vi "TestMain.vi"() -> ()   [LabVIEW 2019]
uses:
  <vilib>/Platform/TimedLoop/XDataNode/timing_clust.ctl
  <vilib>/Platform/TimedLoop/XDataNode/nitl_modes.ctl
  <vilib>/Platform/TimedLoop/XDataNode/wakeup.ctl
  <vilib>/myRIO/Instrument Drivers/Onboard IO/PWM/typedefs/PWM Reference.ctl
  <vilib>/myRIO/Common/Instrument Driver Framework/Utilities/typedefs/myRIO Generic Hardware Reference.ctl
  <vilib>/myRIO/Common/Instrument Driver Framework/Utilities/typedefs/Hardware Version Enum.ctl
  <vilib>/myRIO/Common/Instrument Driver Framework/Utilities/typedefs/myRIO v1.0 Reference.ctl
  <vilib>/myRIO/Common/Instrument Driver Framework/Utilities/typedefs/Generic FPGA Reference.ctl
  <vilib>/myRIO/Common/Instrument Driver Framework/myRIO v1.0/PWM/typedefs/PWM Channels Enum.ctl
  <vilib>/myRIO/Instrument Drivers/Onboard IO/PWM/typedefs/PWM Configuration.ctl
  <vilib>/userdefined/High Color/nirio_resource_hc.ctl
  <vilib>/myRIO/Instrument Drivers/Onboard IO/DIO/typedefs/DIO Reference.ctl
  <vilib>/myRIO/Common/Instrument Driver Framework/myRIO v1.0/DIO/typedefs/DIO Channels List.ctl
  <vilib>/myRIO/Common/Instrument Driver Framework/myRIO v1.0/DIO/typedefs/DIO Channels Enum.ctl
  <vilib>/myRIO/Common/Instrument Driver Framework/Utilities/vis/Is FPGA Ref Available.vi
  <vilib>/myRIO/Common/Instrument Driver Framework/myRIO v1.0/PWM/vis/myRIO v1.1 Open PWM.vi
  <vilib>/myRIO/Instrument Drivers/Onboard IO/PWM/vis/Set Duty Cycle and Frequency.vi
  <vilib>/myRIO/Common/Instrument Driver Framework/myRIO v1.0/DIO/vis/myRIO v1.1 Open DIO.vi
  <extravilib>/ChannelInstances/Tag-bool/Write With Abort.vi
  <extravilib>/ChannelInstances/Tag-bool/Read With Abort.vi
  <vilib>/myRIO/Common/Instrument Driver Framework/Utilities/vis/Validate Channels.vi
  <vilib>/myRIO/Common/Instrument Driver Framework/myRIO v1.0/PWM/vis/myRIO v1.0 Reserve PWM.vi
  <vilib>/myRIO/Common/Instrument Driver Framework/myRIO v1.0/DIO/vis/myRIO v1.0 Reserve DIO.vi
  <vilib>/myRIO/Common/Instrument Driver Framework/myRIO v1.0/I2C/vis/myRIO v1.0 Close I2C.vi
  <vilib>/myRIO/Common/Instrument Driver Framework/myRIO v1.0/UART/vis/myRIO v1.0 Close UART.vi
  <vilib>/myRIO/Common/Instrument Driver Framework/myRIO v1.0/PWM/vis/myRIO v1.0 Build MUX Configuration PWM.vi
  <vilib>/myRIO/Common/Instrument Driver Framework/myRIO v1.0/Resource Manager/vis/myRIO v1.0 Reserve Channel List.vi
  <vilib>/myRIO/Common/Instrument Driver Framework/myRIO v1.0/DIO/vis/myRIO v1.0 Build MUX Configuration DIO.vi
  <vilib>/myRIO/Common/Instrument Driver Framework/myRIO v1.0/I2C/vis/myRIO v1.0 Unreserve I2C.vi
  <vilib>/myRIO/Common/Instrument Driver Framework/myRIO v1.0/Resource Manager/vis/myRIO v1.0 Create Configuration List.vi
  <vilib>/myRIO/Common/Instrument Driver Framework/myRIO v1.0/Resource Manager/vis/myRIO v1.0 Reserve Channel.vi
  <vilib>/myRIO/Common/Instrument Driver Framework/myRIO v1.0/Resource Manager/vis/myRIO v1.0 Unreserve Channel.vi
  <vilib>/myRIO/Common/Instrument Driver Framework/myRIO v1.0/I2C/vis/myRIO v1.0 Build MUX Configuration I2C.vi
  <vilib>/myRIO/Common/Instrument Driver Framework/myRIO v1.0/Resource Manager/vis/myRIO v1.0 Unreserve Channel List.vi
  <vilib>/myRIO/Common/Instrument Driver Framework/myRIO v1.0/Resource Manager/vis/myRIO v1.0 Build Mutex Name.vi
  <vilib>/Instr/_visa.llb/VISA Configure Serial Port (Instr).vi
  <extravilib>/ChannelInstances/Tag-bool/Instantiate.vi
  <extravilib>/ChannelInstances/Tag-bool/EndpointRead.vi
  <vilib>/Utility/VariantDataType/GetNumericInfo.vi
  <vilib>/Utility/error.llb/Error Cluster From Error Code.vi
  <vilib>/myRIO/Common/Instrument Driver Framework/myRIO v1.0/myRIO v1.1 Open.vi
  <vilib>/myRIO/Common/Instrument Driver Framework/Utilities/vis/IO Manager.vi
  <vilib>/myRIO/Common/Instrument Driver Framework/Utilities/vis/Configuration Manager.vi
  <vilib>/myRIO/Common/Instrument Driver Framework/myRIO v1.0/Resource Manager/vis/myRIO v1.0 Configure IO.vi
  <vilib>/myRIO/Common/Instrument Driver Framework/myRIO v1.0/myRIO v1.0 Close.vi
  <vilib>/myRIO/Common/Instrument Driver Framework/myRIO v1.0/PWM/vis/myRIO v1.0 Write PWM.vi
  <vilib>/myRIO/Common/Instrument Driver Framework/myRIO v1.0/DIO/vis/myRIO v1.0 Write DIO.vi
  <vilib>/myRIO/Common/Instrument Driver Framework/myRIO v1.0/I2C/vis/myRIO v1.0 Shutdown I2C.vi
  <vilib>/rvi/errors/niLvFpgaAdjustHostInterfaceError.vi
  <vilib>/FPGAPlugInAG/Dynamic/niLvFpga_Abort_Dynamic.vi
  <vilib>/myRIO/Common/Instrument Driver Framework/Utilities/vis/FPGA Ref Manager.vi
  <vilib>/myRIO/Common/Instrument Driver Framework/myRIO v1.0/myRIO v1.0 Reset FPGA.vi
  <vilib>/myRIO/Common/Instrument Driver Framework/myRIO v1.0/IRQ/vis/myRIO v1.0 IRQ Info FGV.vi
  <vilib>/myRIO/Common/Instrument Driver Framework/myRIO v1.0/IRQ/vis/myRIO v1.0 Timer IRQ Info FGV.vi
  <vilib>/myRIO/Common/Instrument Driver Framework/myRIO v1.0/IRQ/vis/myRIO v1.0 ISR Agent.vi
  <vilib>/myRIO/Instrument Drivers/Utilities/vis/Reset Index.vi
  <vilib>/myRIO/Common/Instrument Driver Framework/myRIO v1.0/Resource Manager/vis/myRIO v1.0 Block Write Resource Manager.vi
  <vilib>/FPGAPlugInAG/Dynamic/niLvFpga_Close_Dynamic.vi
  <extravilib>/ChannelInstances/Tag-bool/Endpoint.vi
  <vilib>/platform/TimedLoop/XDataNode/XDataNode.xnode
  <vilib>/myRIO/Express VI/Onboard IO/PWM/PWM Express VI.xnode
  <vilib>/myRIO/Instrument Drivers/Onboard IO/PWM/vis/myRIO PWM Open.xnode
  <vilib>/myRIO/Express VI/Onboard IO/DO/DO Express VI.xnode
  <vilib>/myRIO/Instrument Drivers/Onboard IO/DIO/vis/myRIO DIO Open.xnode
  <vilib>/rvi/interface/nirviReadWriteControl/nirviReadWriteControl.xnode
  <vilib>/rvi/interface/nirviMethod/nirviMethod.xnode
  <vilib>/rvi/interface/nirviCloseFPGA/nirviCloseFPGA.xnode
  <vilib>/rvi/interface/Simulation/niFpgaSimulationCallBeginRW.vi
  <vilib>/Platform/TimedLoop/XDataNode/XDNodeRunTimeDep.lvlib
  <vilib>/myRIO/Instrument Drivers/Utilities/Utilities.lvlib
  NiFpgaLv.dll
  <extravilib>/ChannelInstances/Tag-bool.lvlib
  <vilib>/myRIO/Instrument Drivers/Onboard IO/PWM/PWM.lvlib
  <vilib>/myRIO/Instrument Drivers/Onboard IO/DIO/DIO.lvlib
  <vilib>/myRIO/Instrument Drivers/Onboard IO/I2C/I2C.lvlib
panel:
  in  "Log file path":path
  out "Duty Cycle":dbl
  in  "Angle limit":i32
  in  "D":dbl
  in  "I":dbl
  in  "P":dbl
  in  "RPM":u16
  out "Raw output from GPS":string
  in  "Organised Output from the GPS":T1(tab)
  out "GPGSV":string
  out "number of message":string
  out "msg1":string
  out "Satelite in view":string
  in  "Satelite_id/elevation/azimuth/SNR 17":enum32{"Msg 1", "Msg 2", "Msg 3", "Msg 4"}(tab)
  out "Satelite_id/elevation/azimuth/SNR":string[](array[string])
  out "Satelite_id/elevation/azimuth/SNR 2":string[](array[string])
  out "Satelite_id/elevation/azimuth/SNR 3":string[](array[string])
  out "Satelite_id/elevation/azimuth/SNR 4":string[](array[string])
  out "Signal ID / Check sum":string[](array[string])
  out "Signal ID / Check sum 2":string[](array[string])
  out "Satelite_id/elevation/azimuth/SNR 8":string[](array[string])
  out "Satelite_id/elevation/azimuth/SNR 7":string[](array[string])
  out "Satelite_id/elevation/azimuth/SNR 6":string[](array[string])
  out "Satelite_id/elevation/azimuth/SNR 5":string[](array[string])
  out "Signal ID / Check sum 3":string[](array[string])
  out "Satelite_id/elevation/azimuth/SNR 12":string[](array[string])
  out "Satelite_id/elevation/azimuth/SNR 11":string[](array[string])
  out "Satelite_id/elevation/azimuth/SNR 10":string[](array[string])
  out "Satelite_id/elevation/azimuth/SNR 9":string[](array[string])
  out "Signal ID / Check sum 4":string[](array[string])
  out "Satelite_id/elevation/azimuth/SNR 16":string[](array[string])
  out "Satelite_id/elevation/azimuth/SNR 15":string[](array[string])
  out "Satelite_id/elevation/azimuth/SNR 14":string[](array[string])
  out "Satelite_id/elevation/azimuth/SNR 13":string[](array[string])
  out "GLGSV 2":string
  out "number of message 2":string
  out "msg1 2":string
  out "Satelite in view 2":string
  in  "Satelite_id/elevation/azimuth/SNR 34":enum32{"Msg 1", "Msg 2", "Msg 3", "Msg 4"}(tab)
  out "Satelite_id/elevation/azimuth/SNR 21":string[](array[string])
  out "Satelite_id/elevation/azimuth/SNR 20":string[](array[string])
  out "Satelite_id/elevation/azimuth/SNR 19":string[](array[string])
  out "Satelite_id/elevation/azimuth/SNR 18":string[](array[string])
  out "Signal ID / Check sum 5":string[](array[string])
  out "Signal ID / Check sum 6":string[](array[string])
  out "Satelite_id/elevation/azimuth/SNR 25":string[](array[string])
  out "Satelite_id/elevation/azimuth/SNR 22":string[](array[string])
  out "Satelite_id/elevation/azimuth/SNR 23":string[](array[string])
  out "Satelite_id/elevation/azimuth/SNR 24":string[](array[string])
  out "Signal ID / Check sum 7":string[](array[string])
  out "Satelite_id/elevation/azimuth/SNR 29":string[](array[string])
  out "Satelite_id/elevation/azimuth/SNR 26":string[](array[string])
  out "Satelite_id/elevation/azimuth/SNR 27":string[](array[string])
  out "Satelite_id/elevation/azimuth/SNR 28":string[](array[string])
  out "Signal ID / Check sum 8":string[](array[string])
  out "Satelite_id/elevation/azimuth/SNR 33":string[](array[string])
  out "Satelite_id/elevation/azimuth/SNR 30":string[](array[string])
  out "Satelite_id/elevation/azimuth/SNR 31":string[](array[string])
  out "Satelite_id/elevation/azimuth/SNR 32":string[](array[string])
  out "GAGSV 3":string
  out "number of message 3":string
  out "msg1 3":string
  out "Satelite in view 3":string
  in  "Satelite_id/elevation/azimuth/SNR 51":enum32{"Msg 1", "Msg 2", "Msg 3", "Msg 4"}(tab)
  out "Satelite_id/elevation/azimuth/SNR 38":string[](array[string])
  out "Satelite_id/elevation/azimuth/SNR 37":string[](array[string])
  out "Satelite_id/elevation/azimuth/SNR 36":string[](array[string])
  out "Satelite_id/elevation/azimuth/SNR 35":string[](array[string])
  out "Signal ID / Check sum 9":string[](array[string])
  out "Signal ID / Check sum 10":string[](array[string])
  out "Satelite_id/elevation/azimuth/SNR 42":string[](array[string])
  out "Satelite_id/elevation/azimuth/SNR 39":string[](array[string])
  out "Satelite_id/elevation/azimuth/SNR 40":string[](array[string])
  out "Satelite_id/elevation/azimuth/SNR 41":string[](array[string])
  out "Signal ID / Check sum 11":string[](array[string])
  out "Satelite_id/elevation/azimuth/SNR 46":string[](array[string])
  out "Satelite_id/elevation/azimuth/SNR 43":string[](array[string])
  out "Satelite_id/elevation/azimuth/SNR 44":string[](array[string])
  out "Satelite_id/elevation/azimuth/SNR 45":string[](array[string])
  out "Signal ID / Check sum 12":string[](array[string])
  out "Satelite_id/elevation/azimuth/SNR 50":string[](array[string])
  out "Satelite_id/elevation/azimuth/SNR 47":string[](array[string])
  out "Satelite_id/elevation/azimuth/SNR 48":string[](array[string])
  out "Satelite_id/elevation/azimuth/SNR 49":string[](array[string])
  out "GBGSV 4":string
  out "number of message 4":string
  out "msg1 4":string
  out "Satelite in view 4":string
  in  "Satelite_id/elevation/azimuth/SNR 68":enum32{"Msg 1", "Msg 2", "Msg 3", "Msg 4"}(tab)
  out "Satelite_id/elevation/azimuth/SNR 55":string[](array[string])
  out "Satelite_id/elevation/azimuth/SNR 54":string[](array[string])
  out "Satelite_id/elevation/azimuth/SNR 53":string[](array[string])
  out "Satelite_id/elevation/azimuth/SNR 52":string[](array[string])
  out "Signal ID / Check sum 13":string[](array[string])
  out "Signal ID / Check sum 14":string[](array[string])
  out "Satelite_id/elevation/azimuth/SNR 59":string[](array[string])
  out "Satelite_id/elevation/azimuth/SNR 56":string[](array[string])
  out "Satelite_id/elevation/azimuth/SNR 57":string[](array[string])
  out "Satelite_id/elevation/azimuth/SNR 58":string[](array[string])
  out "Signal ID / Check sum 15":string[](array[string])
  out "Satelite_id/elevation/azimuth/SNR 63":string[](array[string])
  out "Satelite_id/elevation/azimuth/SNR 60":string[](array[string])
  out "Satelite_id/elevation/azimuth/SNR 61":string[](array[string])
  out "Satelite_id/elevation/azimuth/SNR 62":string[](array[string])
  out "Signal ID / Check sum 16":string[](array[string])
  out "Satelite_id/elevation/azimuth/SNR 67":string[](array[string])
  out "Satelite_id/elevation/azimuth/SNR 64":string[](array[string])
  out "Satelite_id/elevation/azimuth/SNR 65":string[](array[string])
  out "Satelite_id/elevation/azimuth/SNR 66":string[](array[string])
  out "UTC Time":string
  out "N/S":string
  out "Long":string
  out "Mode":string
  out "Status":string
  out "Lat":string
  out "Course over Ground [Degrees]":string
  out "date[ddmmyy]":string
  out "E/W":string
  out "Speed over ground[knot]":string
  out "xxRMC":string
  out "NavStatus":string
  out "Checksum":string
  out "Carriage return":string
  out "Lat 2":string
  out "NS":string
  out "GLL":string
  out "Long 3":string
  out "EW":string
  out "Time":string
  out "Status 2":string
  out "Positioning mod":string
  out "Check sum":string
  out "Carriage return 2":string
  out "VTG":string
  out "Course over Ground":string
  out "Reference":string
  out "Course over Ground (Magnetic)":string
  out "Reference2":string
  out "Speedover Ground (knots)":string
  out "Units1":string
  out "Speed over ground kph":string
  out "Units 2":string
  out "Position Mode 2":string
  out "Check sum 2":string
  out "GGA 3":string
  out "UTC time":string
  out "Lat 3":string
  out "NS 2":string
  out "Long 2":string
  out "EW 2":string
  out "Pos_indicator":string
  out "Number of Satelite_used":string
  out "hdop":string
  out "msl_altitude":string
  out "altitude_units":string
  out "geoidal_Seperation":string
  out "Separation unit":string
  out "age of Diff corr":string
  out "diffStating":string
  out "Checksum 2":string
  out "GSA":string
  out "Operation Mode":string
  out "Navigation mode":string
  out "satelite used channel 1":string
  out "satelite used channel 3":string
  out "satelite used channel 4":string
  out "satelite used channel 5":string
  out "satelite used channel 6":string
  out "satelite used channel 7":string
  out "satelite used channel 8":string
  out "satelite used channel 9":string
  out "satelite used channel 10":string
  out "satelite used channel 11":string
  out "satelite used channel 12":string
  out "pdop":string
  out "hdop 2":string
  out "vdop":string
  out "System ID":string
  out "Checksum 3":string
  out "satelite used channel 2":string
  out "Combined loop duration time (us)":i64
  in  "Loop durations":T2(tab)
  out "IMU Data gathering duration(us)":i64(graph)
  out "Hall data gathering duration(us)":i64(graph)
  out "Encoder data gathering duration(us)":i64(graph)
  out "Steering Motor duration(us)":i64(graph)
  out "E-Stop loop duration (us)":i64(graph)
  out "GPS loop duration (us)":i64(graph)
  in  "GO":bool
  in  "E-stop":bool
  out "Indicator":bool
  in  "Encoder Position Reset":bool
  out "Encoder Velocity (Counts/Interval)":i32
  out "Encoder Acceleration (Counts/Interval)":i32
  out "Encoder Position (Counts)":i32
  out "Hall Detection":bool
  out "Hall Period":u32
  out "IMU Gyro Chart":cluster{dbl, dbl, dbl}(graph)
  out "IMU Acc Chart":cluster{dbl, dbl, dbl}(graph)
  # "Steering Motor"
  # "Forward Motor"
  # "Start Motors"
  # "Signal ID / Check sum"
  # "Signal ID / Check sum"
  # "Signal ID / Check sum"
  # "Signal ID / Check sum"
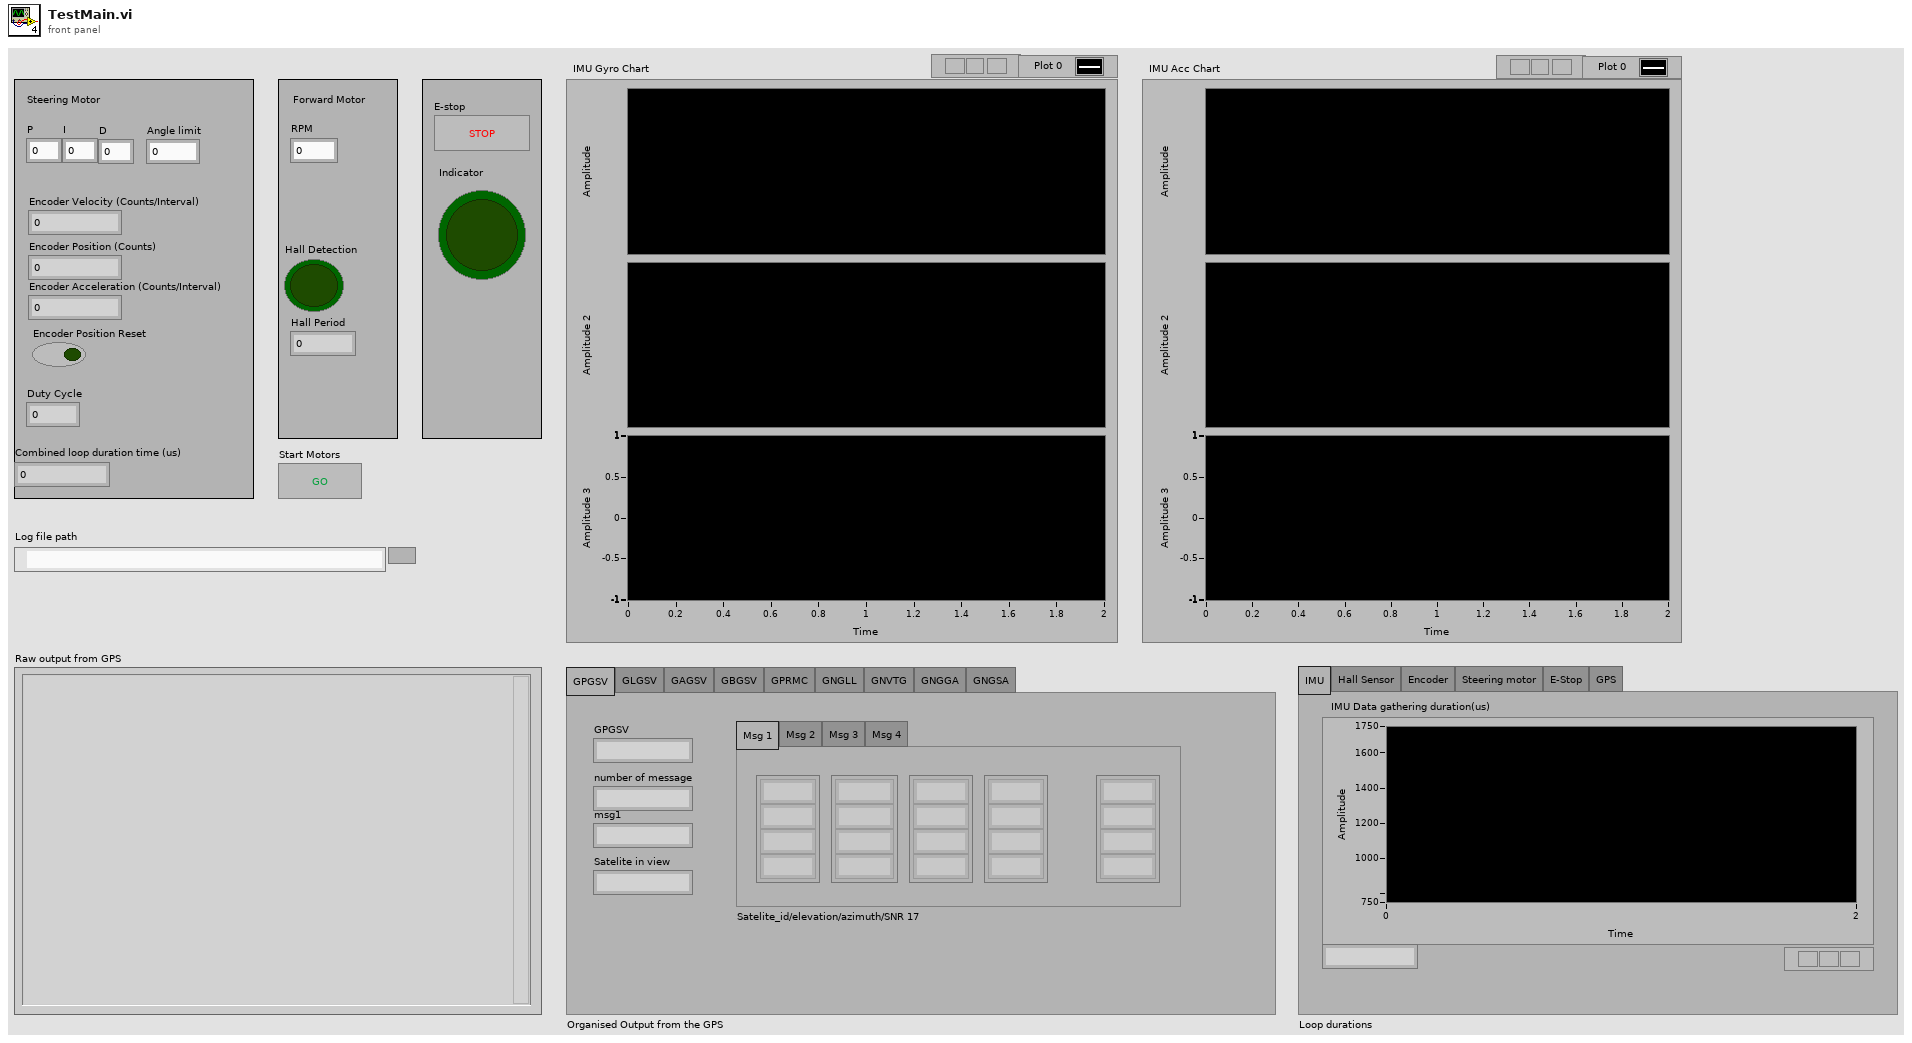
[diagram p1: front panel]
types:
  T1 = enum32{"GPGSV", "GLGSV", "GAGSV", "GBGSV", "GPRMC", "GNGLL", "GNVTG", "GNGGA", "GNGSA"}
  T2 = enum32{"IMU", "Hall Sensor", "Encoder", "Steering motor", "E-Stop", "GPS"}
  T3 = enum16{"open", "open or create", "create or replace", "create", "open (read-only)"}
  T4 = typedef "I2C.lvlib/I2C Reference.ctl" = cluster{"myRIO Reference":T5, "I2C Channels Enum":T9, "I2C Configuration":T10}
  T5 = typedef "myRIO Generic Hardware Reference.ctl" = cluster{"myRIO Model":T6, "myRIO Hardware Reference":T7}
  T6 = typedef "Hardware Version Enum.ctl" = enum16{"Unknown", "myRIO-1900", "myRIO-1950", "roboRIO", "NI ELVIS RIO CM", "ELVIS III"}
  T7 = typedef "myRIO v1.0 Reference.ctl" = cluster{"Generic FPGA Reference":T8, "Allow multiple opens":bool}
  T8 = typedef "Generic FPGA Reference.ctl" = refnum<k20>
  T9 = typedef "I2C Channels Enum.ctl" = enum16{"Not Connected", "A/I2C", "B/I2C", "I2C/I2C"}
  T10 = typedef "I2C.lvlib/I2C Configuration.ctl" = cluster{"I2C Transfer Rate":T11}
  T11 = typedef "I2C.lvlib/I2C Transfer Rate.ctl" = enum16{"Standard mode (100 kbps)", "Fast mode (400 kbps)"}
  T12 = typedef "XDNodeRunTimeDep.lvlib/timing_clust.ctl" = cluster{"Expected End [f-1]":u64, "Actual End [f-1]":u64, "Finished Late? [f-1]":bool, "Expected End [i-1]":u64, "Actual End [i-1]":u64, "Finished Late? [i-1]":bool, "Expected Start [i]":u64, "Actual Start [i]":u64, "Expected Start [f]":u64, "Actual Start [f]":u64, "Source Name":string, "Structure Name":string, "Period":i64, "Deadline":i64, "Offset":i64, "Start":i64, "Priority":i32, "Timeout":i32, "Mode":T13, "Wakeup Reason":T14, "Error":errorcluster, "Source Type":string, "Secondary Source Type":string, "Global End Time":u64, "Global Start Time":u64, "Frame Duration":u64, "Iteration Duration":u64, "Assigned CPU":i32, "I/O Scan Engine Mode":u32}
  T13 = typedef "XDNodeRunTimeDep.lvlib/nitl_modes.ctl" = enum32{"No Change", "Process missed periods, maintain original phase", "Discard missed periods, maintain original phase", "Process missed periods, ignore original phase", "Discard missed periods, ignore original phase"}
  T14 = typedef "XDNodeRunTimeDep.lvlib/wakeup.ctl" = enum32{"Normal", "Aborted", "Asynchronous wakeup", "Timing source error", "Timed loop error", "Timeout"}
  T15 = typedef "Tag-bool.lvlib/))Channel.ctl" = refnum<queue>
  T16 = typedef "PWM.lvlib/PWM Reference.ctl" = cluster{"myRIO Reference":T5, "PWM Channels Enum":T17, "PWM Configuration":T18}
  T17 = typedef "PWM Channels Enum.ctl" = enum16{"Not Connected", "C/PWM0", "C/PWM1", "A/PWM0", "A/PWM1", "A/PWM2", "A/PWM3", "A/PWM4", "A/PWM5", "A/PWM6", "A/PWM7", "A/PWM8", "A/PWM9", "A/PWM10", "A/PWM11", "A/PWM12", "A/PWM13", "A/PWM14", "A/PWM15", "A/PWM16", "A/PWM17", "A/PWM18", "A/PWM19", "B/PWM0", "B/PWM1", "B/PWM2", "B/PWM3", "B/PWM4", "B/PWM5", "B/PWM6", "B/PWM7", "B/PWM8", "B/PWM9", "B/PWM10", "B/PWM11", "B/PWM12", "B/PWM13", "B/PWM14", "B/PWM15", "B/PWM16", "B/PWM17", "B/PWM18", "B/PWM19", "PWM/PWM0", "PWM/PWM1", "PWM/PWM2", "PWM/PWM3", "PWM/PWM4", "PWM/PWM5", "PWM/PWM6", "PWM/PWM7", "PWM/PWM8", "PWM/PWM9"}
  T18 = typedef "PWM.lvlib/PWM Configuration.ctl" = cluster{"Frequency":dbl, "Duty Cycle":dbl}
  T19 = typedef "nirio_resource_hc.ctl" = tag
  T20 = typedef "DIO.lvlib/DIO Reference.ctl" = cluster{"myRIO Reference":T5, "DIO Channels List":T21}
  T21 = typedef "DIO Channels List.ctl" = T22[]
  T22 = typedef "DIO Channels Enum.ctl" = enum16{"Not Connected", "C/DIO0", "C/DIO1", "C/DIO2", "C/DIO3", "C/DIO4", "C/DIO5", "C/DIO6", "C/DIO7", "A/DIO0", "A/DIO1", "A/DIO2", "A/DIO3", "A/DIO4", "A/DIO5", "A/DIO6", "A/DIO7", "A/DIO8", "A/DIO9", "A/DIO10", "A/DIO11", "A/DIO12", "A/DIO13", "A/DIO14", "A/DIO15", "A/DIO16", "A/DIO17", "A/DIO18", "A/DIO19", "B/DIO0", "B/DIO1", "B/DIO2", "B/DIO3", "B/DIO4", "B/DIO5", "B/DIO6", "B/DIO7", "B/DIO8", "B/DIO9", "B/DIO10", "B/DIO11", "B/DIO12", "B/DIO13", "B/DIO14", "B/DIO15", "B/DIO16", "B/DIO17", "B/DIO18", "B/DIO19", "LED0", "LED1", "LED2", "LED3", "Button0", "DIO/DIO0", "DIO/DIO1", "DIO/DIO2", "DIO/DIO3", "DIO/DIO4", "DIO/DIO5", "DIO/DIO6", "DIO/DIO7", "DIO/DIO8", "DIO/DIO9", "SPI/CS0", "SPI/CS1", "SPI/CS2", "SPI/CS3", "LED RADIO (Green)", "LED RADIO (Red)", "LED COMM (Green)", "LED COMM (Red)", "LED MODE (Green)", "LED MODE (Red)"}
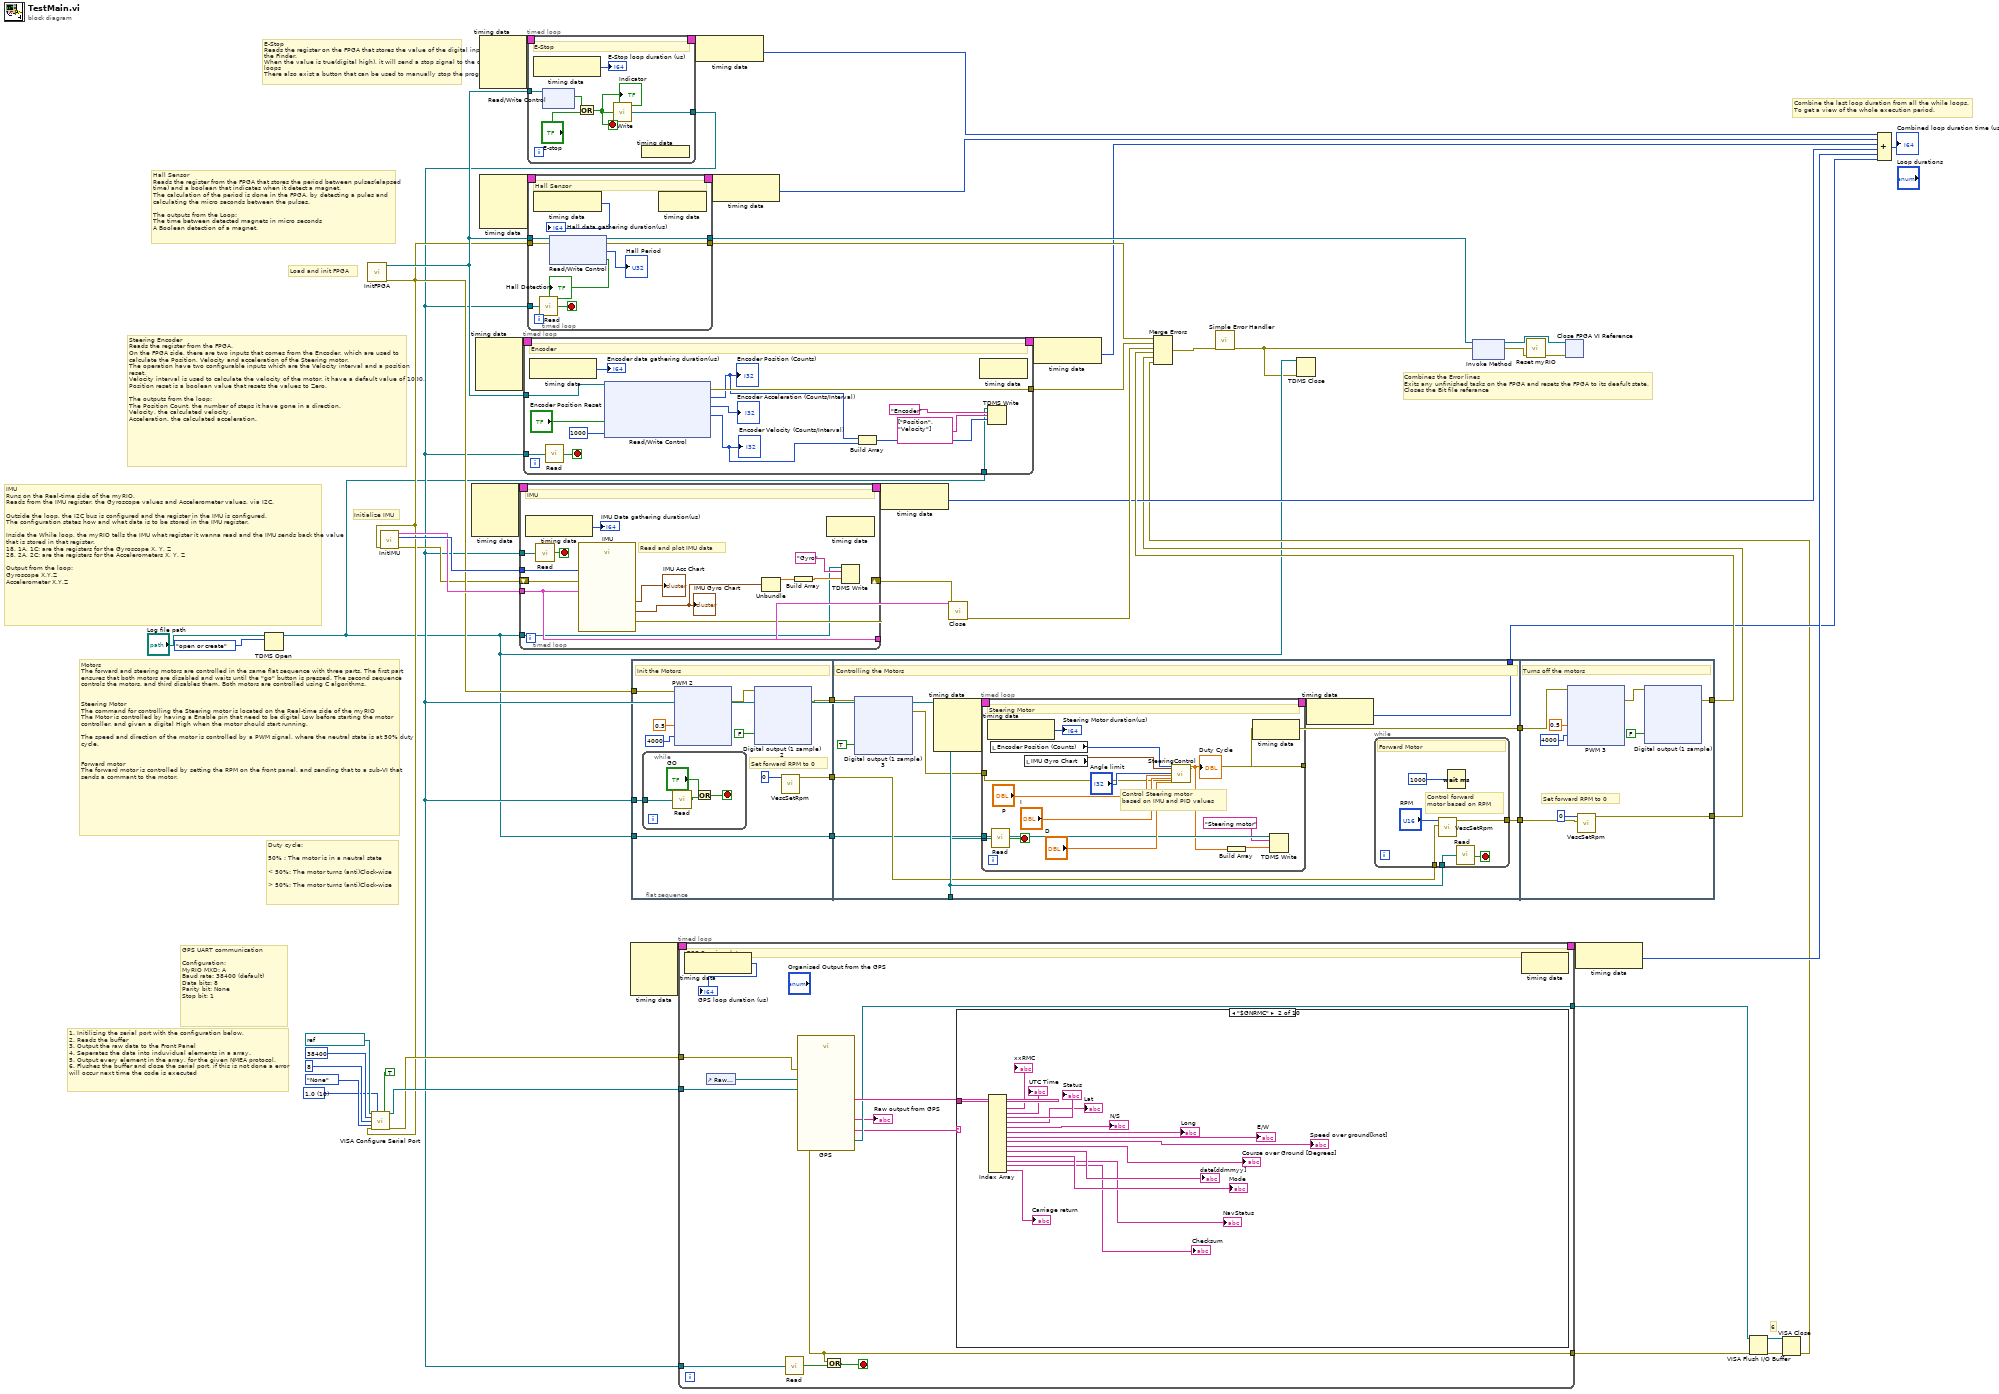
[diagram p0: block diagram]
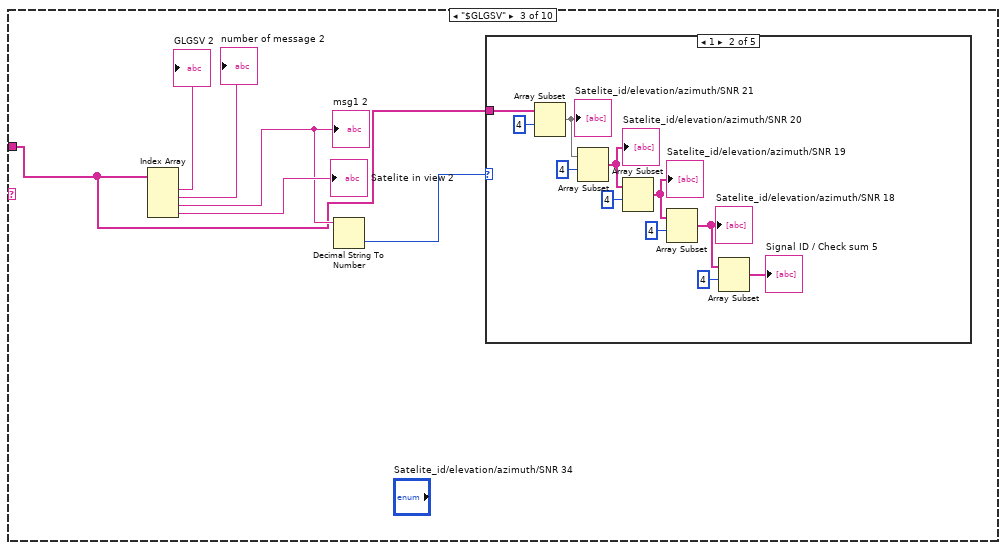
[diagram p3: hidden frame]
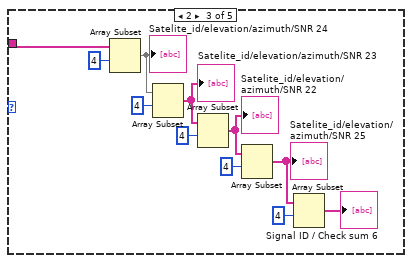
[diagram p5: hidden frame]
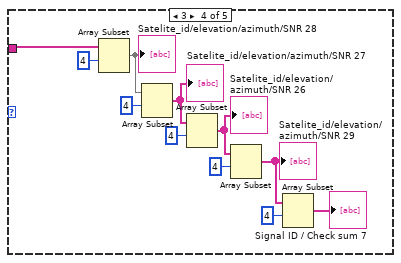
[diagram p6: hidden frame]
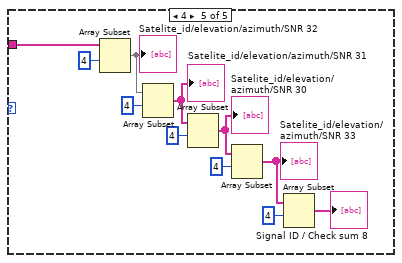
[diagram p7: hidden frame]
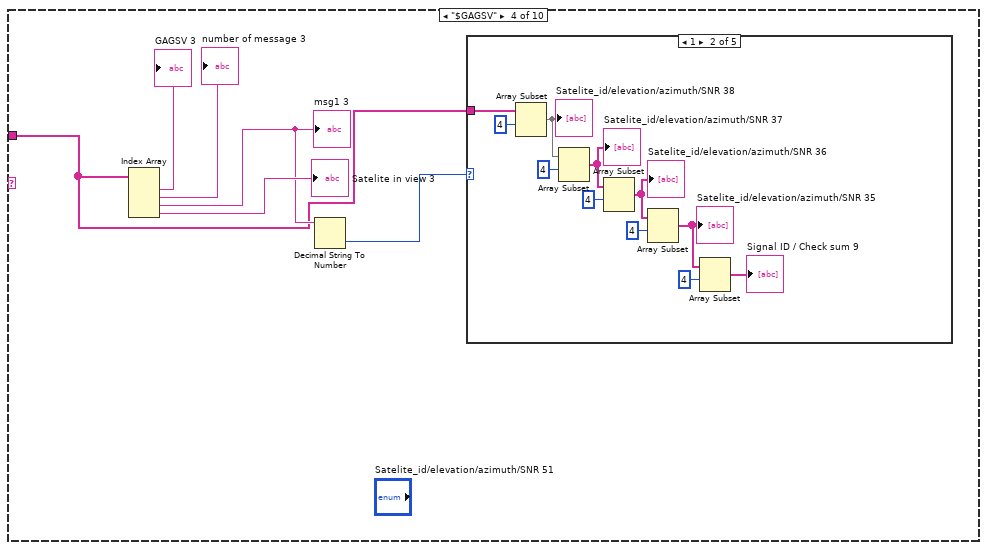
[diagram p8: hidden frame]
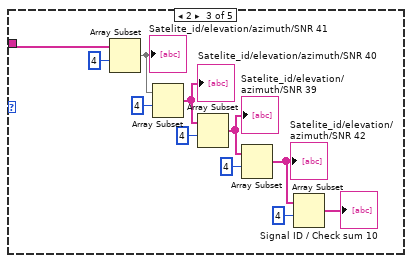
[diagram p10: hidden frame]
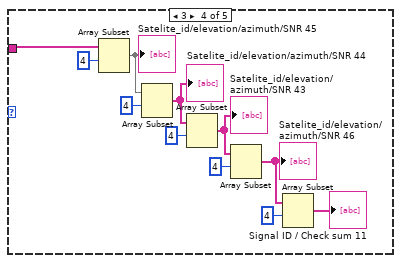
[diagram p11: hidden frame]
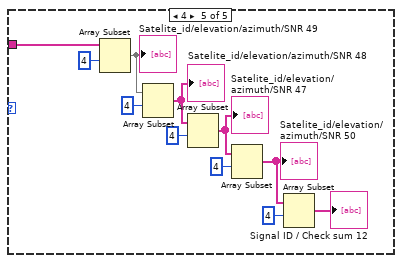
[diagram p12: hidden frame]
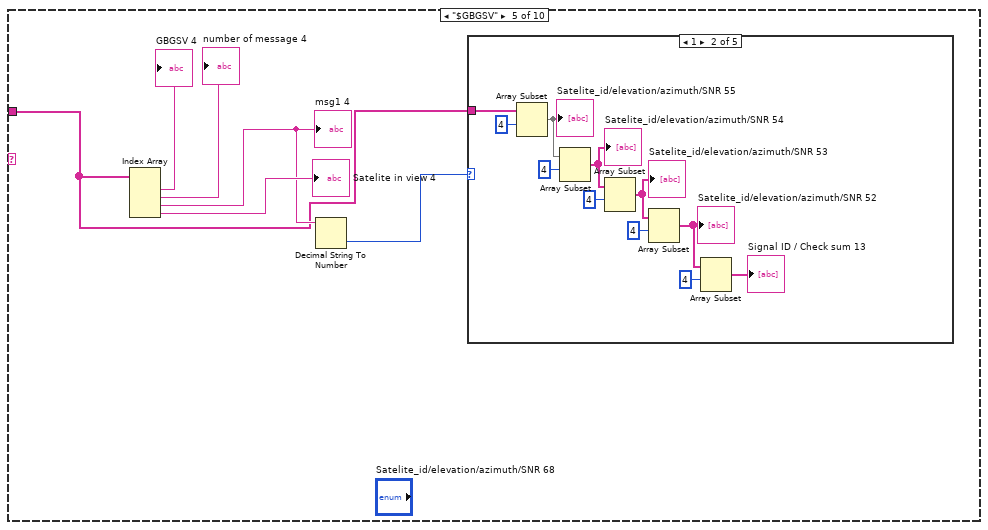
[diagram p13: hidden frame]
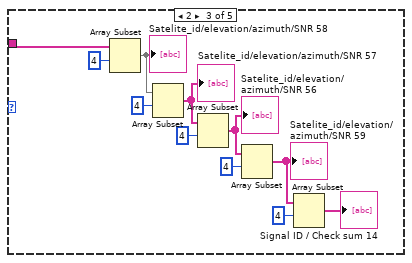
[diagram p15: hidden frame]
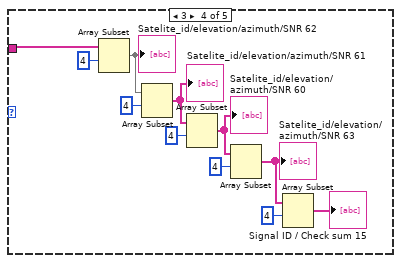
[diagram p16: hidden frame]
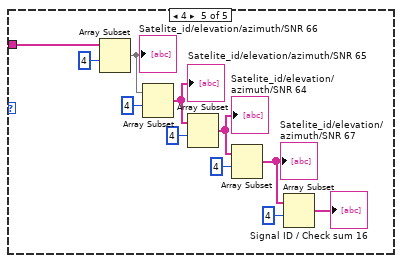
[diagram p17: hidden frame]
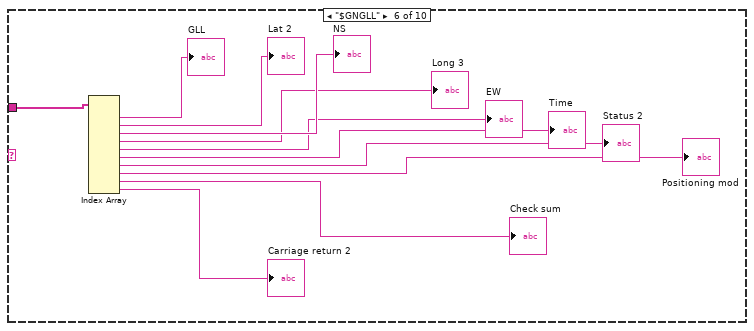
[diagram p18: hidden frame]
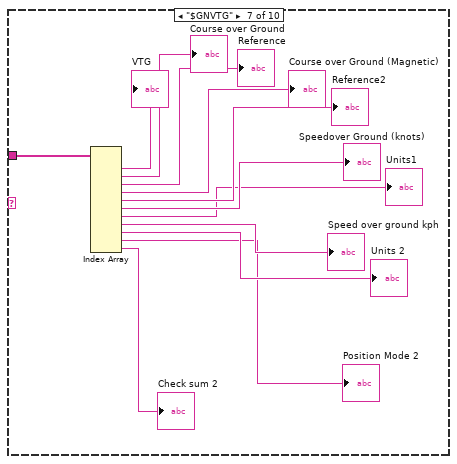
[diagram p19: hidden frame]
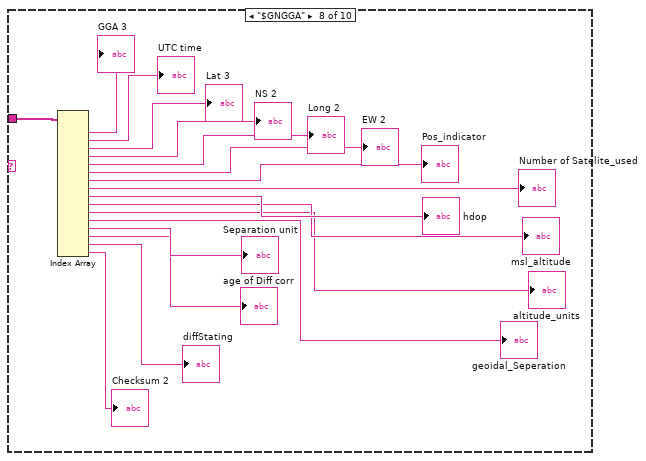
[diagram p20: hidden frame]
diagram:
  w27 = u16 10 items=["1.0"=10, "1.5"=15, "2.0"=20] ("stop bits (10: 1 bit)")
  # "Duty cycle:\n\n50% : The motor is in a neutral state\n\n< 50%: The motor turns (anti)Clock-wise\n\n> 50%: The motor turns (anti)Clock-wise"
  # "Initialize IMU"
  # "Load and init FPGA"
  # "Combines the Error lines\nExits any unfinished tasks on the FPGA and resets the FPGA to its deafult state.\nCloses the Bit file referance"
  # "Combine the last loop duration from all the while loops.\nTo get a view of the whole execution period."
  # "1. Initilizing the serial port with the configuration below.\n2. Reads the buffer\n3. Output the raw data to the Front Panel\n4. Seperates the data into induvidual elements in a array.\n5. Output every element in the array, for the given NMEA protocol.\n6. Flushes the buffer and close the serial port, if this is not done a error will occur next time the code is executed"
  # "Motors\nThe forward and steering motors are controlled in the same flat sequence with three parts. The first part ensures that both motors are disabled and waits until the \"go\" button is pressed. The second sequence controls the motors, and third disables them. Both motors are controlled using C algorithms.\n\n\nSteering Motor\nThe command for controlling the Steering motor is located on the Real-time side of the myRIO\nThe Motor is controlled by having a Enable pin that need to be digital Low before starting the motor controller, and given a digital High when the motor should start running.\n\nThe speed and direction of the motor is controlled by a PWM signal, where the neutral state is at 50% duty cycle.\n\n\nForward motor\nThe forward motor is controlled by setting the RPM on the front panel, and sending that to a sub-VI that sends a commant to the motor."
  # "IMU\nRuns on the Real-time side of the myRIO.\nReads from the IMU register, the Gyroscope values and Accelerometer values, via I2C.\n\nOutside the loop, the I2C bus is configured and the register in the IMU is configured.\nThe configuration states how and what data is to be stored in the IMU register.\n\nInside the While loop, the myRIO tells the IMU what register it wanna read and the IMU sends back the value that is stored in that register.\n18, 1A, 1C: are the registers for the Gyroscope X, Y, Z\n28, 2A, 2C: are the registers for the Accelerometers X, Y, Z\n\nOutput from the loop:\nGyroscope X,Y,Z\nAccelerometer X,Y,Z"
  # "Steering Encoder\nReads the register from the FPGA. \nOn the FPGA side, there are two inputs that comes from the Encoder, which are used to calculate the Position, Velocity and acceleration of the Steering motor.\nThe operation have two configurable inputs which are the Velocity interval and a position reset.\nVelocity interval is used to calculate the velocity of the motor, it have a default value of 1000.\nPosition reset is a boolean value that resets the values to Zero.\n\nThe outputs from the loop:\nThe Position Count, the number of steps it have gone in a direction. \nVelocity, the calculated velocity.\nAcceleration, the calculated acceleration."
  # "Hall Sensor\nReads the register from the FPGA that stores the period between pulses(elapsed time) and a boolean that indicates when it detect a magnet.\nThe calculation of the period is done in the FPGA, by detecting a pules and calculating the micro seconds between the pulses.\n\nThe outputs from the Loop:\nThe time between detected magnets in micro seconds\nA Boolean detection of a magnet."
  # "E-Stop\nReads the register on the FPGA that stores the value of the digital input from the Finder.\nWhen the value is true(digital high), it will send a stop signal to the other while loops\nThere also exist a button that can be used to manually stop the program."
  # "6"
  # "GPS UART communication\n\nConfiguration:\nMyRIO MXD: A\nBaud rate: 38400 (default)\nData bits: 8\nParity bit: None\nStop bit: 1"
  n1 = TDMS Open(10:T3."open or create" ("operation (0:open)"), 11:"Log file path") -> (3:w2:refnum<k34>)  [unwired: 5 in, 1 out]
  n2 = call "InitFPGA.vi"() -> ("error out"=w21:errorcluster, "Refnum out"=w35:refnum<k20>)  [unwired: 10 in]
  n3 = call-poly "VISA Configure Serial Port"("VISA resource name"=refnum<visa-resource-name> "ASRL1::INSTR", "Enable Termination\nChar (T)"=TRUE ("Enable Termination\nChar (T)"), "baud rate (9600)"=u32 38400, "data bits (8)"=u16 8, "parity (0:none)"=enum16{"None", "Odd", "Even", "Mark", "Space"}."None", "error in (no error)"=w21, "stop bits (10: 1 bit)"=w27) -> ("VISA resource name out"=w24:refnum<visa-resource-name>, "error out"=w23:errorcluster)  [unwired: 7 in]
  n4 = call "InitIMU.vi"("error in (no error)"=w21) -> ("error out"=w15:errorcluster, "Acc/Gyro  address"=w37:u8, "I2C Ref Out"=w36:T4)  [unwired: 8 in]
  n5 = node-c288() -> (w46:T12)  [unwired: 4 in]
  n6 = node-c288() -> (w51:T12)  [unwired: 4 in]
  n7 = node-c288() -> (w44:T12)  [unwired: 4 in]
  n8 = node-c288() -> (w53:T12)  [unwired: 4 in]
  n9 = timed-loop {
    timing: w44 -> [_]
    timing-out: [_] -> w43
    tunnel: w35 -> [w63]
    tunnel: [w62] -> w11
    stop <- w58 stop-if-true
    # "E-Stop"
    n10 = node-c288() -> (→"E-Stop loop duration (us)":i64)  [unwired: 1 in]
    n11 = xnode "Read/Write Control"("FPGA VI Reference In"=w63) -> ("E-Stop"=w61:bool)  [unwired: 1 in, 2 out]
    n12 = Or(x=w61, y="E-stop") -> (x .or. y?=w58:bool)
    "Indicator" <- w58
    n13 = call <vilib>:"Write.vi"("element"=w58) -> ("channel"=w62:T15)  [unwired: 1 out]
    n14 = node-c288() -> ()  [unwired: 1 out]
  }
  n15 = timed-loop {
    timing: w46 -> [_]
    timing-out: [_] -> w45
    tunnel: w37 -> [w79]
    tunnel: w36 -> [w76]
    shift-right: [w72] -> w16
    shift-left: w15 -> [w78]
    tunnel: [w76] -> w20
    tunnel: w11 -> [w75]
    tunnel: w2 -> [w67]
    stop <- w74 stop-if-true
    # "Read and plot IMU data"
    # "IMU"
    n16 = node-c288() -> (→"IMU Data gathering duration(us)":i64)  [unwired: 1 in]
    n17 = call <extravilib>:"Read.vi"("channel"=w75) -> ("element"=w74:bool)  [unwired: 1 in, 1 out]
    n18 = call "IMU.vi"("error in (no error)"=w78, "Acc/Gyro  address"=w79, "I2C Ref"=w76) -> ("error out"=w72:errorcluster, "IMU Acc"=→"IMU Acc Chart":cluster{dbl, dbl, dbl}, "IMU Gyro"=w71:cluster{dbl, dbl, dbl})  [unwired: 6 in]
    "IMU Gyro Chart" <- w71
    n19 = Unbundle(w71) -> (w70:dbl)  [unwired: 2 out]
    n20 = Build Array(w70) -> (w68:dbl[])
    n21 = node-c288() -> ()  [unwired: 1 in, 1 out]
    n22 = TDMS Write(0:w67, 5:"Gyro" ("group name in (Untitled)"), 9:w68) -> ()  [unwired: 3 in, 4 out]
  }
  n23 = timed-loop {
    timing: w51 -> [_]
    timing-out: [_] -> w50
    tunnel: w35 -> [w96]
    tunnel: [w95] -> w48
    tunnel: w11 -> [w90]
    tunnel: w2 -> [w83]
    stop <- w89 stop-if-true
    # "Encoder"
    n24 = node-c288() -> (→"Encoder data gathering duration(us)":i64)  [unwired: 1 in]
    n25 = call <extravilib>:"Read.vi"("channel"=w90) -> ("element"=w89:bool)  [unwired: 1 in, 1 out]
    n26 = xnode "Read/Write Control"("FPGA VI Reference In"=w96, "Position Reset"="Encoder Position Reset", "Velocity Interval (uSec)"=u32 1000) -> ("error out"=w95:errorcluster, "Position (Counts)"=w86:i32, "Acceleration (Counts/Interval)"=→"Encoder Acceleration (Counts/Interval)":i32, "Velocity (Counts/Interval)"=w85:i32)  [unwired: 1 in, 1 out]
    "Encoder Position (Counts)" <- w86
    "Encoder Velocity (Counts/Interval)" <- w85
    n27 = Build Array(w86, w85) -> (w84:i32[])
    n28 = node-c288() -> ()  [unwired: 1 in, 1 out]
    n29 = TDMS Write(0:w83, 5:"Encoder" ("group name in (Untitled)"), 7:string[] ["Position", "Velocity"] ("channel name(s) in (Untitled)"), 9:w84) -> ()  [unwired: 2 in, 4 out]
  }
  n30 = timed-loop {
    tunnel: w21 -> [w108]
    tunnel: w35 -> [w107]
    tunnel: [w105] -> w54
    tunnel: [w104] -> w49
    timing: w53 -> [_]
    timing-out: [_] -> w52
    tunnel: w11 -> [w101]
    stop <- w100 stop-if-true
    # "Hall Sensor"
    n31 = node-c288() -> (→"Hall data gathering duration(us)":i64)  [unwired: 1 in]
    n32 = call <extravilib>:"Read.vi"("channel"=w101) -> ("element"=w100:bool)  [unwired: 1 in, 1 out]
    n33 = xnode "Read/Write Control"("FPGA VI Reference In"=w107, "error in"=w108) -> ("FPGA VI Reference Out"=w105:refnum<k20>, "error out"=w104:errorcluster, "Hall Period"=→"Hall Period":u32, "Hall Detection"=→"Hall Detection":bool)
    n34 = node-c288() -> ()  [unwired: 1 in, 1 out]
  }
  n35 = node-c288() -> (w34:T12)  [unwired: 4 in]
  n36 = flat-sequence {
    tunnel: [w120] -> w42
    tunnel: w21 -> [w118]
    tunnel: w11 -> [w114]
    tunnel: [w113] -> w10
    tunnel: w2 -> [w112]
    tunnel: [w112] -> w3
    tunnel: w42 -> [w206]
    tunnel: [w203] -> w12
    tunnel: w11 -> [w200]
    tunnel: w10 -> [w199]
    tunnel: [w198] -> w9
    tunnel: [w197] -> w6
    tunnel: w3 -> [w196]
    tunnel: [w276] -> w17
    tunnel: w9 -> [w271]
    tunnel: [w270] -> w7
    tunnel: w6 -> [w269]
    frame #0 {
      # "Set forward RPM to 0"
      # "Init the Motors"
      n37 = while {
        tunnel: w114 -> [w122]
        stop <- w125 stop-if-true
        n38 = call <extravilib>:"Read.vi"("channel"=w122) -> ("element"=w123:bool)  [unwired: 1 in, 1 out]
        n39 = Or(x="GO", y=w123) -> (x .or. y?=w125:bool)
      }
      n40 = xnode "PWM 2"("Duty Cycle"=0.5, "Frequency [Hz]"=4000, "error in (no error)"=w118) -> ("error out"=w121:errorcluster)
      n41 = xnode "Digital output (1 sample) 2"("B/DIO4 (Pin 19)"=FALSE ("B/DIO1 (Pin 13)"), "error in (no error)"=w121) -> ("error out"=w120:errorcluster)
      n42 = call "VescSetRpm.vi"("RPM"=0) -> ("error out"=w113:errorcluster)  [unwired: 10 in]
    }
    frame #1 {
      # "Controlling the Motors"
      n43 = xnode "Digital output (1 sample) 3"("B/DIO4 (Pin 19)"=TRUE ("B/DIO1 (Pin 13)"), "error in (no error)"=w206) -> ("error out"=w202:errorcluster)
      n44 = node-c288() -> (w205:T12)  [unwired: 4 in]
      n45 = timed-loop {
        tunnel: w202 -> [w218]
        timing: w205 -> [_]
        timing-out: [_] -> w204
        tunnel: w200 -> [w220]
        tunnel: [w217] -> w197
        tunnel: w196 -> [w216]
        stop <- w227 stop-if-true
        # "Control Steering motor\nbased on IMU and PID values"
        # "Steering Motor"
        n46 = node-c288() -> (→"Steering Motor duration(us)":i64)  [unwired: 1 in]
        n47 = local read "Encoder Position (Counts)"() -> (w224:i32)
        n48 = call <extravilib>:"Read.vi"("channel"=w220) -> ("element"=w227:bool)  [unwired: 1 in, 1 out]
        n49 = local read "IMU Gyro Chart"() -> (w225:cluster{dbl, dbl, dbl})
        n50 = call "SteeringControl.vi"("Position (Counts)"=w224, "Cluster"=w225, "Limit"="Angle limit", "P gain"="P", "I gain"="I", "error in (no error)"=w218, "D gain"="D") -> ("error out"=w217:errorcluster, "PWM Out"=w213:dbl)  [unwired: 19 in]
        "Duty Cycle" <- w213
        n51 = Build Array(w213) -> (w214:dbl[])
        n52 = node-c288() -> ()  [unwired: 1 in, 1 out]
        n53 = TDMS Write(0:w216, 5:"Steering motor" ("group name in (Untitled)"), 9:w214) -> ()  [unwired: 3 in, 4 out]
      }
      n54 = node-c288(w204) -> (w203:i64)
      n55 = while "Timed Loop" {
        tunnel: w200 -> [w210]
        tunnel: w199 -> [w208]
        tunnel: [w207] -> w198
        stop <- w211 stop-if-true
        # "Control forward\nmotor based on RPM"
        # "Forward Motor"
        n56 = call "VescSetRpm.vi"("error in (no error)"=w208, "RPM"="RPM") -> ("error out"=w207:errorcluster)  [unwired: 9 in]
        n57 = Wait (ms)(milliseconds to wait=1000) -> ()  [unwired: 1 out]
        n58 = call <extravilib>:"Read.vi"("channel"=w210) -> ("element"=w211:bool)  [unwired: 1 in, 1 out]
      }
    }
    frame #2 {
      # "Set forward RPM to 0"
      # "Turns off the motors"
      n59 = xnode "PWM 3"("Duty Cycle"=0.5, "Frequency [Hz]"=4000, "error in (no error)"=w269) -> ("error out"=w273:errorcluster)
      n60 = call "VescSetRpm.vi"("error in (no error)"=w271, "RPM"=0) -> ("error out"=w270:errorcluster)  [unwired: 9 in]
      n61 = xnode "Digital output (1 sample)"("B/DIO4 (Pin 19)"=FALSE ("B/DIO1 (Pin 13)"), "error in (no error)"=w273) -> ("error out"=w276:errorcluster)
    }
  }
  n62 = timed-loop {
    tunnel: [w358] -> w19
    tunnel: w24 -> [w357]
    tunnel: w23 -> [w356]
    tunnel: [w354] -> w22
    timing: w34 -> [_]
    timing-out: [_] -> w33
    tunnel: w11 -> [w352]
    stop <- w355 stop-if-true
    # "GPS Receive data"
    n63 = node-c288() -> (→"GPS loop duration (us)":i64)  [unwired: 1 in]
    n64 = control-ref of="Raw output from GPS"() -> (w350:refnum<vi>)
    n65 = call <extravilib>:"Read.vi"("channel"=w352) -> ("element"=w351:bool)  [unwired: 1 in, 1 out]
    n66 = call "GPS.vi"("error in (no error)"=w356, "reference"=w350, "VISA Refnum"=w357) -> ("error out"=w354:errorcluster, "Array"=w359:string[], "Raw output from GPS"=→"Raw output from GPS":string, "VISA Refnum"=w358:refnum<visa-resource-name>, "read buffer"=w348:string)  [unwired: 4 in]
    n67 = Or(x=w354, y=w351) -> (x .or. y?=w355:bool)
    n68 = case shown="\"$GNRMC\"" w348 {
      tunnel: w359 -> [_ w377 w378 w428 w478 w538 w550 w567 w588 w589]
      frame "False", Default {
      }
      frame "$GNRMC" {
        n69 = Index Array(array=w377) -> (element #1=→"xxRMC":string, element #2=→"UTC Time":string, element #3=→"Status":string, element #4=→"Lat":string, element #5=→"N/S":string, element #6=→"Long":string, element #7=→"E/W":string, element #8=→"Speed over ground[knot]":string, element #9=→"Course over Ground [Degrees]":string, element #10=→"date[ddmmyy]":string, element #11=→"Mode":string, element #12=→"NavStatus":string, element #13=→"Checksum":string, element #14=→"Carriage return":string)  [unwired: 14 in]
      }
      frame "$GLGSV" {
        n70 = Index Array(array=w378) -> (element #1=→"GLGSV 2":string, element #2=→"number of message 2":string, element #3=w380:string, element #4=→"Satelite in view 2":string)  [unwired: 4 in]
        "msg1 2" <- w380
        n71 = Decimal String To Number(string=w380) -> (number=w379:i32)  [unwired: 2 in, 1 out]
        n72 = case shown="1" w379 {
          tunnel: w378 -> [_ w385 w395 w406 w417]
          frame 0, Default {
          }
          frame 1 {
            n73 = Array Subset(array=w385, index=4) -> (w390:string[])  [unwired: 1 in]
            "Satelite_id/elevation/azimuth/SNR 21" <- w390
            n74 = Array Subset(array=w390, index=4) -> (w391:string[])  [unwired: 1 in]
            "Satelite_id/elevation/azimuth/SNR 20" <- w391
            n75 = Array Subset(array=w391, index=4) -> (w392:string[])  [unwired: 1 in]
            "Satelite_id/elevation/azimuth/SNR 19" <- w392
            n76 = Array Subset(array=w392, index=4) -> (w394:string[])  [unwired: 1 in]
            "Satelite_id/elevation/azimuth/SNR 18" <- w394
            n77 = Array Subset(array=w394, index=4) -> (→"Signal ID / Check sum 5":string[])  [unwired: 1 in]
          }
          frame 2 {
            n78 = Array Subset(array=w395, index=4) -> (w401:string[])  [unwired: 1 in]
            "Satelite_id/elevation/azimuth/SNR 24" <- w401
            n79 = Array Subset(array=w401, index=4) -> (w402:string[])  [unwired: 1 in]
            "Satelite_id/elevation/azimuth/SNR 23" <- w402
            n80 = Array Subset(array=w402, index=4) -> (w403:string[])  [unwired: 1 in]
            "Satelite_id/elevation/azimuth/SNR 22" <- w403
            n81 = Array Subset(array=w403, index=4) -> (w405:string[])  [unwired: 1 in]
            "Satelite_id/elevation/azimuth/SNR 25" <- w405
            n82 = Array Subset(array=w405, index=4) -> (→"Signal ID / Check sum 6":string[])  [unwired: 1 in]
          }
          frame 3 {
            n83 = Array Subset(array=w406, index=4) -> (w412:string[])  [unwired: 1 in]
            "Satelite_id/elevation/azimuth/SNR 28" <- w412
            n84 = Array Subset(array=w412, index=4) -> (w413:string[])  [unwired: 1 in]
            "Satelite_id/elevation/azimuth/SNR 27" <- w413
            n85 = Array Subset(array=w413, index=4) -> (w414:string[])  [unwired: 1 in]
            "Satelite_id/elevation/azimuth/SNR 26" <- w414
            n86 = Array Subset(array=w414, index=4) -> (w416:string[])  [unwired: 1 in]
            "Satelite_id/elevation/azimuth/SNR 29" <- w416
            n87 = Array Subset(array=w416, index=4) -> (→"Signal ID / Check sum 7":string[])  [unwired: 1 in]
          }
          frame 4 {
            n88 = Array Subset(array=w417, index=4) -> (w423:string[])  [unwired: 1 in]
            "Satelite_id/elevation/azimuth/SNR 32" <- w423
            n89 = Array Subset(array=w423, index=4) -> (w424:string[])  [unwired: 1 in]
            "Satelite_id/elevation/azimuth/SNR 31" <- w424
            n90 = Array Subset(array=w424, index=4) -> (w425:string[])  [unwired: 1 in]
            "Satelite_id/elevation/azimuth/SNR 30" <- w425
            n91 = Array Subset(array=w425, index=4) -> (w427:string[])  [unwired: 1 in]
            "Satelite_id/elevation/azimuth/SNR 33" <- w427
            n92 = Array Subset(array=w427, index=4) -> (→"Signal ID / Check sum 8":string[])  [unwired: 1 in]
          }
        }
      }
      frame "$GAGSV" {
        n93 = Index Array(array=w428) -> (element #1=→"GAGSV 3":string, element #2=→"number of message 3":string, element #3=w430:string, element #4=→"Satelite in view 3":string)  [unwired: 4 in]
        "msg1 3" <- w430
        n94 = Decimal String To Number(string=w430) -> (number=w429:i32)  [unwired: 2 in, 1 out]
        n95 = case shown="1" w429 {
          tunnel: w428 -> [_ w435 w445 w456 w467]
          frame 0, Default {
          }
          frame 1 {
            n96 = Array Subset(array=w435, index=4) -> (w440:string[])  [unwired: 1 in]
            "Satelite_id/elevation/azimuth/SNR 38" <- w440
            n97 = Array Subset(array=w440, index=4) -> (w441:string[])  [unwired: 1 in]
            "Satelite_id/elevation/azimuth/SNR 37" <- w441
            n98 = Array Subset(array=w441, index=4) -> (w442:string[])  [unwired: 1 in]
            "Satelite_id/elevation/azimuth/SNR 36" <- w442
            n99 = Array Subset(array=w442, index=4) -> (w444:string[])  [unwired: 1 in]
            "Satelite_id/elevation/azimuth/SNR 35" <- w444
            n100 = Array Subset(array=w444, index=4) -> (→"Signal ID / Check sum 9":string[])  [unwired: 1 in]
          }
          frame 2 {
            n101 = Array Subset(array=w445, index=4) -> (w451:string[])  [unwired: 1 in]
            "Satelite_id/elevation/azimuth/SNR 41" <- w451
            n102 = Array Subset(array=w451, index=4) -> (w452:string[])  [unwired: 1 in]
            "Satelite_id/elevation/azimuth/SNR 40" <- w452
            n103 = Array Subset(array=w452, index=4) -> (w453:string[])  [unwired: 1 in]
            "Satelite_id/elevation/azimuth/SNR 39" <- w453
            n104 = Array Subset(array=w453, index=4) -> (w455:string[])  [unwired: 1 in]
            "Satelite_id/elevation/azimuth/SNR 42" <- w455
            n105 = Array Subset(array=w455, index=4) -> (→"Signal ID / Check sum 10":string[])  [unwired: 1 in]
          }
          frame 3 {
            n106 = Array Subset(array=w456, index=4) -> (w462:string[])  [unwired: 1 in]
            "Satelite_id/elevation/azimuth/SNR 45" <- w462
            n107 = Array Subset(array=w462, index=4) -> (w463:string[])  [unwired: 1 in]
            "Satelite_id/elevation/azimuth/SNR 44" <- w463
            n108 = Array Subset(array=w463, index=4) -> (w464:string[])  [unwired: 1 in]
            "Satelite_id/elevation/azimuth/SNR 43" <- w464
            n109 = Array Subset(array=w464, index=4) -> (w466:string[])  [unwired: 1 in]
            "Satelite_id/elevation/azimuth/SNR 46" <- w466
            n110 = Array Subset(array=w466, index=4) -> (→"Signal ID / Check sum 11":string[])  [unwired: 1 in]
          }
          frame 4 {
            n111 = Array Subset(array=w467, index=4) -> (w473:string[])  [unwired: 1 in]
            "Satelite_id/elevation/azimuth/SNR 49" <- w473
            n112 = Array Subset(array=w473, index=4) -> (w474:string[])  [unwired: 1 in]
            "Satelite_id/elevation/azimuth/SNR 48" <- w474
            n113 = Array Subset(array=w474, index=4) -> (w475:string[])  [unwired: 1 in]
            "Satelite_id/elevation/azimuth/SNR 47" <- w475
            n114 = Array Subset(array=w475, index=4) -> (w477:string[])  [unwired: 1 in]
            "Satelite_id/elevation/azimuth/SNR 50" <- w477
            n115 = Array Subset(array=w477, index=4) -> (→"Signal ID / Check sum 12":string[])  [unwired: 1 in]
          }
        }
      }
      frame "$GBGSV" {
        n116 = Index Array(array=w478) -> (element #1=→"GBGSV 4":string, element #2=→"number of message 4":string, element #3=w480:string, element #4=→"Satelite in view 4":string)  [unwired: 4 in]
        "msg1 4" <- w480
        n117 = Decimal String To Number(string=w480) -> (number=w479:i32)  [unwired: 2 in, 1 out]
        n118 = case shown="1" w479 {
          tunnel: w478 -> [_ w485 w495 w506 w517]
          frame 0, Default {
          }
          frame 1 {
            n119 = Array Subset(array=w485, index=4) -> (w490:string[])  [unwired: 1 in]
            "Satelite_id/elevation/azimuth/SNR 55" <- w490
            n120 = Array Subset(array=w490, index=4) -> (w491:string[])  [unwired: 1 in]
            "Satelite_id/elevation/azimuth/SNR 54" <- w491
            n121 = Array Subset(array=w491, index=4) -> (w492:string[])  [unwired: 1 in]
            "Satelite_id/elevation/azimuth/SNR 53" <- w492
            n122 = Array Subset(array=w492, index=4) -> (w494:string[])  [unwired: 1 in]
            "Satelite_id/elevation/azimuth/SNR 52" <- w494
            n123 = Array Subset(array=w494, index=4) -> (→"Signal ID / Check sum 13":string[])  [unwired: 1 in]
          }
          frame 2 {
            n124 = Array Subset(array=w495, index=4) -> (w501:string[])  [unwired: 1 in]
            "Satelite_id/elevation/azimuth/SNR 58" <- w501
            n125 = Array Subset(array=w501, index=4) -> (w502:string[])  [unwired: 1 in]
            "Satelite_id/elevation/azimuth/SNR 57" <- w502
            n126 = Array Subset(array=w502, index=4) -> (w503:string[])  [unwired: 1 in]
            "Satelite_id/elevation/azimuth/SNR 56" <- w503
            n127 = Array Subset(array=w503, index=4) -> (w505:string[])  [unwired: 1 in]
            "Satelite_id/elevation/azimuth/SNR 59" <- w505
            n128 = Array Subset(array=w505, index=4) -> (→"Signal ID / Check sum 14":string[])  [unwired: 1 in]
          }
          frame 3 {
            n129 = Array Subset(array=w506, index=4) -> (w512:string[])  [unwired: 1 in]
            "Satelite_id/elevation/azimuth/SNR 62" <- w512
            n130 = Array Subset(array=w512, index=4) -> (w513:string[])  [unwired: 1 in]
            "Satelite_id/elevation/azimuth/SNR 61" <- w513
            n131 = Array Subset(array=w513, index=4) -> (w514:string[])  [unwired: 1 in]
            "Satelite_id/elevation/azimuth/SNR 60" <- w514
            n132 = Array Subset(array=w514, index=4) -> (w516:string[])  [unwired: 1 in]
            "Satelite_id/elevation/azimuth/SNR 63" <- w516
            n133 = Array Subset(array=w516, index=4) -> (→"Signal ID / Check sum 15":string[])  [unwired: 1 in]
          }
          frame 4 {
            n134 = Array Subset(array=w517, index=4) -> (w523:string[])  [unwired: 1 in]
            "Satelite_id/elevation/azimuth/SNR 66" <- w523
            n135 = Array Subset(array=w523, index=4) -> (w524:string[])  [unwired: 1 in]
            "Satelite_id/elevation/azimuth/SNR 65" <- w524
            n136 = Array Subset(array=w524, index=4) -> (w525:string[])  [unwired: 1 in]
            "Satelite_id/elevation/azimuth/SNR 64" <- w525
            n137 = Array Subset(array=w525, index=4) -> (w527:string[])  [unwired: 1 in]
            "Satelite_id/elevation/azimuth/SNR 67" <- w527
            n138 = Array Subset(array=w527, index=4) -> (→"Signal ID / Check sum 16":string[])  [unwired: 1 in]
          }
        }
      }
      frame "$GNGLL" {
        n139 = Index Array(array=w538) -> (element #1=→"GLL":string, element #2=→"Lat 2":string, element #3=→"NS":string, element #4=→"Long 3":string, element #5=→"EW":string, element #6=→"Time":string, element #7=→"Status 2":string, element #8=→"Positioning mod":string, element #9=→"Check sum":string, element #10=→"Carriage return 2":string)  [unwired: 10 in]
      }
      frame "$GNVTG" {
        n140 = Index Array(array=w550) -> (element #1=→"VTG":string, element #2=→"Course over Ground":string, element #3=→"Reference":string, element #4=→"Course over Ground (Magnetic)":string, element #5=→"Reference2":string, element #6=→"Speedover Ground (knots)":string, element #7=→"Units1":string, element #8=→"Speed over ground kph":string, element #9=→"Units 2":string, element #10=→"Position Mode 2":string, element #11=→"Check sum 2":string)  [unwired: 11 in]
      }
      frame "$GNGGA" {
        n141 = Index Array(array=w567) -> (element #1=→"GGA 3":string, element #2=→"UTC time":string, element #3=→"Lat 3":string, element #4=→"NS 2":string, element #5=→"Long 2":string, element #6=→"EW 2":string, element #7=→"Pos_indicator":string, element #8=→"Number of Satelite_used":string, element #9=→"hdop":string, element #10=→"msl_altitude":string, element #11=→"altitude_units":string, element #12=→"geoidal_Seperation":string, element #13=→"Separation unit":string, element #14=→"age of Diff corr":string, element #15=→"diffStating":string, element #16=→"Checksum 2":string)  [unwired: 16 in]
      }
      frame "$GNGSA" {
        n142 = Index Array(array=w588) -> (element #1=→"GSA":string, element #2=→"Operation Mode":string, element #3=→"Navigation mode":string, element #4=→"satelite used channel 1":string, element #5=→"satelite used channel 2":string, element #6=→"satelite used channel 3":string, element #7=→"satelite used channel 4":string, element #8=→"satelite used channel 5":string, element #9=→"satelite used channel 6":string, element #10=→"satelite used channel 7":string, element #11=→"satelite used channel 8":string, element #12=→"satelite used channel 9":string, element #13=→"satelite used channel 10":string, element #14=→"satelite used channel 11":string, element #15=→"satelite used channel 12":string, element #16=→"pdop":string, element #17=→"hdop 2":string, element #18=→"vdop":string, element #19=→"System ID":string, element #20=→"Checksum 3":string)  [unwired: 20 in]
      }
      frame "$GPGSV" {
        n143 = Index Array(array=w589) -> (element #1=→"GPGSV":string, element #2=→"number of message":string, element #3=w591:string, element #4=→"Satelite in view":string)  [unwired: 4 in]
        "msg1" <- w591
        n144 = Decimal String To Number(string=w591) -> (number=w590:i32)  [unwired: 2 in, 1 out]
        n145 = case shown="1" w590 {
          tunnel: w589 -> [_ w596 w606 w617 w628]
          frame 0, Default {
          }
          frame 1 {
            n146 = Array Subset(array=w596, index=4) -> (w601:string[])  [unwired: 1 in]
            "Satelite_id/elevation/azimuth/SNR" <- w601
            n147 = Array Subset(array=w601, index=4) -> (w602:string[])  [unwired: 1 in]
            "Satelite_id/elevation/azimuth/SNR 2" <- w602
            n148 = Array Subset(array=w602, index=4) -> (w603:string[])  [unwired: 1 in]
            "Satelite_id/elevation/azimuth/SNR 3" <- w603
            n149 = Array Subset(array=w603, index=4) -> (w605:string[])  [unwired: 1 in]
            "Satelite_id/elevation/azimuth/SNR 4" <- w605
            n150 = Array Subset(array=w605, index=4) -> (→"Signal ID / Check sum":string[])  [unwired: 1 in]
          }
          frame 2 {
            n151 = Array Subset(array=w606, index=4) -> (w612:string[])  [unwired: 1 in]
            "Satelite_id/elevation/azimuth/SNR 5" <- w612
            n152 = Array Subset(array=w612, index=4) -> (w613:string[])  [unwired: 1 in]
            "Satelite_id/elevation/azimuth/SNR 6" <- w613
            n153 = Array Subset(array=w613, index=4) -> (w614:string[])  [unwired: 1 in]
            "Satelite_id/elevation/azimuth/SNR 7" <- w614
            n154 = Array Subset(array=w614, index=4) -> (w616:string[])  [unwired: 1 in]
            "Satelite_id/elevation/azimuth/SNR 8" <- w616
            n155 = Array Subset(array=w616, index=4) -> (→"Signal ID / Check sum 2":string[])  [unwired: 1 in]
          }
          frame 3 {
            n156 = Array Subset(array=w617, index=4) -> (w623:string[])  [unwired: 1 in]
            "Satelite_id/elevation/azimuth/SNR 9" <- w623
            n157 = Array Subset(array=w623, index=4) -> (w624:string[])  [unwired: 1 in]
            "Satelite_id/elevation/azimuth/SNR 10" <- w624
            n158 = Array Subset(array=w624, index=4) -> (w625:string[])  [unwired: 1 in]
            "Satelite_id/elevation/azimuth/SNR 11" <- w625
            n159 = Array Subset(array=w625, index=4) -> (w627:string[])  [unwired: 1 in]
            "Satelite_id/elevation/azimuth/SNR 12" <- w627
            n160 = Array Subset(array=w627, index=4) -> (→"Signal ID / Check sum 3":string[])  [unwired: 1 in]
          }
          frame 4 {
            n161 = Array Subset(array=w628, index=4) -> (w634:string[])  [unwired: 1 in]
            "Satelite_id/elevation/azimuth/SNR 13" <- w634
            n162 = Array Subset(array=w634, index=4) -> (w635:string[])  [unwired: 1 in]
            "Satelite_id/elevation/azimuth/SNR 14" <- w635
            n163 = Array Subset(array=w635, index=4) -> (w636:string[])  [unwired: 1 in]
            "Satelite_id/elevation/azimuth/SNR 15" <- w636
            n164 = Array Subset(array=w636, index=4) -> (w638:string[])  [unwired: 1 in]
            "Satelite_id/elevation/azimuth/SNR 16" <- w638
            n165 = Array Subset(array=w638, index=4) -> (→"Signal ID / Check sum 4":string[])  [unwired: 1 in]
          }
        }
      }
    }
    n166 = node-c288() -> ()  [unwired: 1 in, 1 out]
  }
  n167 = node-c288(w43) -> (w41:i64)
  n168 = node-c288(w52) -> (w40:i64)
  n169 = node-c288(w45) -> (w14:i64)
  n170 = call <vilib>:"Close.vi"("error in (no error)"=w16, "I2C Ref In"=w20) -> ("error out"=w18:errorcluster)  [unwired: 9 in]
  n171 = node-c288(w50) -> (w39:i64)
  n172 = node-c288(w33) -> (w13:i64)
  n173 = VISA Flush I/O Buffer(VISA resource name=w19, error in (no error)=w22) -> (VISA resource name out=w26:refnum<visa-resource-name>, error out=w25:errorcluster)  [unwired: 1 in]
  n174 = VISA Close(VISA resource name=w26, error in (no error)=w25) -> (error out=w8:errorcluster)
  n175 = Merge Errors(w49, w48, w18, w17, w7, w8) -> (w47:errorcluster)
  n176 = call <vilib>:"Simple Error Handler.vi"("error in (no error)"=w47) -> ("error out"=w1:errorcluster)  [unwired: 4 in, 4 out]
  n177 = TDMS Close(8:w1, 11:w2) -> ()  [unwired: 2 out]
  n178 = xnode "Invoke Method"("FPGA VI Reference In"=w54, "error in"=w1) -> ("FPGA VI Reference Out"=w57:refnum<k20>, "error out"=w55:errorcluster)
  n179 = call <vilib>:"Reset myRIO.vi"("error in (no error)"=w55) -> ("error out"=w56:errorcluster)  [unwired: 10 in]
  n180 = xnode "Close FPGA VI Reference"("FPGA VI Reference In"=w57, "error in"=w56) -> ()  [unwired: 1 out]
  n181 = Compound Arithmetic op=ADD(w41, w40, w39, w14, w13, w12) -> (→"Combined loop duration time (us)":i64)
